vi "Расшифровка слова данных (SubVI).vi"(11 "СД":bool[](array[boolean])) -> (0 "СД верно":bool, 3 "Data":u16 format="%x")   [LabVIEW 2015]
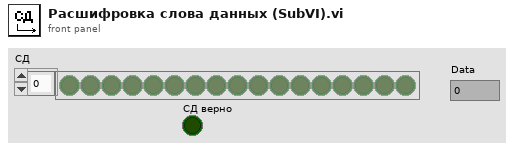
[diagram p1: front panel]
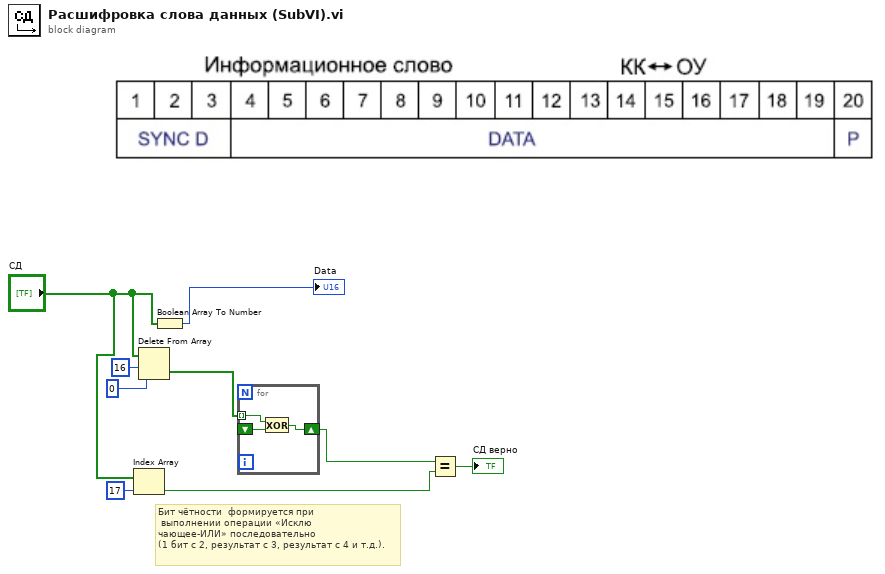
[diagram p0: block diagram]
diagram:
  # "Бит чётности  формируется при\n выполнении операции «Исклю\nчающее-ИЛИ» последовательно \n(1 бит с 2, результат с 3, результат с 4 и т.д.)."
  n1 = Index Array(array="СД", index=17) -> (element=w3:bool)
  n2 = Delete From Array(array="СД", length=16, index=0) -> (deleted portion=w6:bool[])  [unwired: 1 out]
  n3 = Boolean Array To Number(Boolean array="СД") -> (number=→"Data":u32)
  n4 = for {
    tunnel: w6 -> [w12] mode=indexing
    shift-right: [w11] -> w2
    shift-left: _ -> [w10]
    n5 = Exclusive Or(1:w10, 2:w12) -> (0:w11:bool)
  }
  n6 = Equal?(x=w2, y=w3) -> (x = y?=→"СД верно":bool)
